vi "Obtain Static (Named SEQ).vi"(8 "error in (no error)":errorcluster, 11 "Numeric in":refnum<class "Numeric Test Object.lvclass">) -> (0 "error out":errorcluster, 3 "Numeric out":refnum<class "Numeric Test Object.lvclass">)   [LabVIEW 2009, in "Numeric Test Object.lvclass"]
doc: "Obtains a reference to a named SEQ and stores it in the class cluster."
uses:
  Numeric Test Object.lvclass
  Numeric Test Object.lvclass/Numeric Test Object.ctl
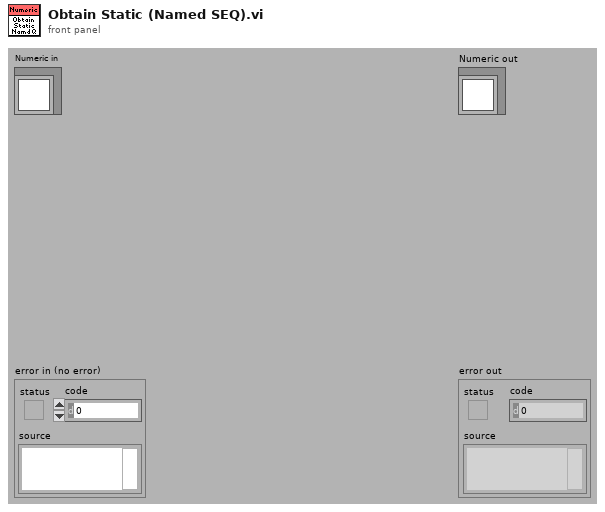
[diagram p1: front panel]
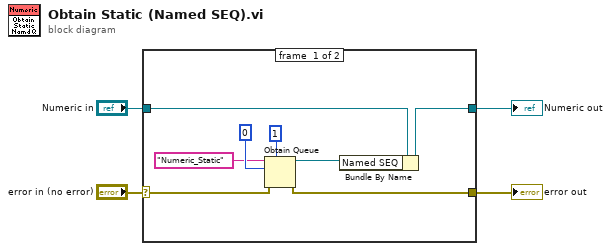
[diagram p0: block diagram]
diagram:
  n1 = case shown="No Error" "error in (no error)" {
    selector: "error in (no error)" -> [w11 w14]
    tunnel: [w6 w14] -> w3
    tunnel: [w12 w13] -> w1
    tunnel: "Numeric in" -> [w8 w13]
    frame #0 {
      n2 = Obtain Queue(max queue size (-1, unlimited)=1, name (unnamed)="Numeric_Static", element data type=0, error in (no error)=w11) -> (queue out=w7:refnum<queue>, error out=w6:errorcluster)  [unwired: 1 in, 1 out]
      n3 = Bundle By Name(cluster=w8, "Named SEQ"=w7) -> (w12:refnum<class "Numeric Test Object.lvclass">)
    }
    frame #1 {
    }
  }
  "error out" <- w3
  "Numeric out" <- w1
